vi "Index.vi"(11 "Index?":bool) -> ()   [LabVIEW 2016]
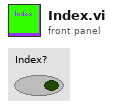
[diagram p1: front panel]
types:
  T1 = typedef "WPI_MotorControlDeviceRef.ctl" = cluster{"DeviceStatus":errorcluster, "Type":T2, "PWM":cluster{"PWM Channel":T3, "DeadBand":T4}, "CAN":cluster{"Device Number":u8, "SetOutput VI Ref":variant, "GetOutput VI Ref":variant, "Enable VI Ref":variant, "Disable VI Ref":variant, "Data":variant}, "Invert":bool}
  T2 = typedef "WPI_MotorControlType.ctl" = enum16{"PWM", "CAN"}
  T3 = typedef "FPGA_DIOPWMChannel.ctl" = enum8{"PWM 0", "PWM 1", "PWM 2", "PWM 3", "PWM 4", "PWM 5", "PWM 6", "PWM 7", "PWM 8", "PWM 9", "PWM MXP 0", "PWM MXP 1", "PWM MXP 2", "PWM MXP 3", "PWM MXP 4", "PWM MXP 5", "PWM MXP 6", "PWM MXP 7", "PWM MXP 8", "PWM MXP 9", "Invalid"}
  T4 = typedef "WPI_PWMDeadband.ctl" = cluster{"Name":string, "maxPositivePwm":i32, "minPositivePwm":i32, "centerPwm":i32, "maxNegativePwm":i32, "minNegativePwm":i32, "angularRange":u16}
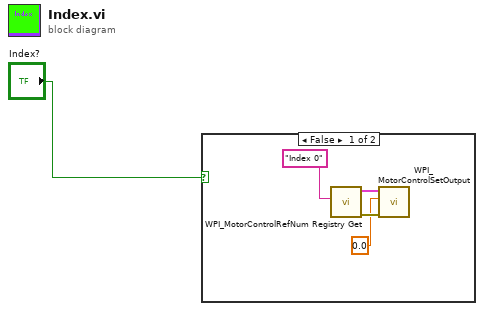
[diagram p0: block diagram]
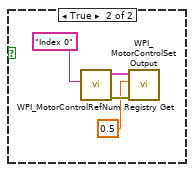
[diagram p2: hidden frame]
diagram:
  n1 = case shown="False" "Index?" {
    frame False {
      n2 = call <vilib>:"WPI_MotorControlRefNum Registry Get.vi"("refnum name"="Index 0") -> ("error out"=w4:errorcluster, "MotorControlDevRef"=w3:T1)  [unwired: 9 in]
      n3 = call <vilib>:"WPI_MotorControlSetOutput.vi"("error in (no error)"=w4, "Output"=0.0, "MotorControlDevRef"=w3) -> ()  [unwired: 6 in, 3 out]
    }
    frame True {
      n4 = call <vilib>:"WPI_MotorControlRefNum Registry Get.vi"("refnum name"="Index 0") -> ("error out"=w8:errorcluster, "MotorControlDevRef"=w7:T1)  [unwired: 9 in]
      n5 = call <vilib>:"WPI_MotorControlSetOutput.vi"("error in (no error)"=w8, "Output"=0.5, "MotorControlDevRef"=w7) -> ()  [unwired: 6 in, 3 out]
    }
  }
